vi "rvc Generate Linear Segment with Parabolic Blend.vi"(7 "maximum velocity":dbl=nan, 9 "number of timesteps":dbl, 10 "final position":dbl, 11 "initial position":dbl) -> (0 "error out":errorcluster, 1 "accelaration":cluster{"time":dbl[], "velocity":dbl[]}(graph), 2 "velocity":cluster{"time":dbl[], "velocity":dbl[]}(graph), 3 "position":cluster{"time":dbl[], "position":dbl[]}(graph))   [LabVIEW 2019]
uses:
  <vilib>/Analysis/1siggen.llb/Ramp Pattern by Samples.vi
  <vilib>/Utility/error.llb/Error Cluster From Error Code.vi
  <vilib>/ErrorRing/Error Ring.xnode
  <vilib>/Analysis/NI_AALBase.lvlib
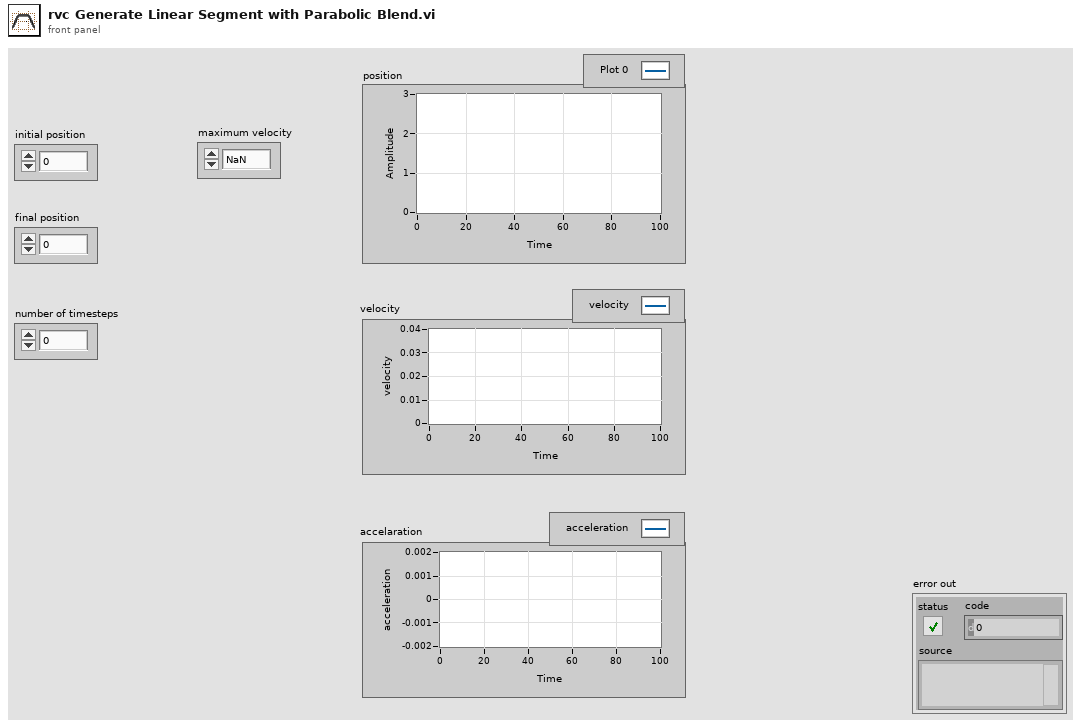
[diagram p1: front panel]
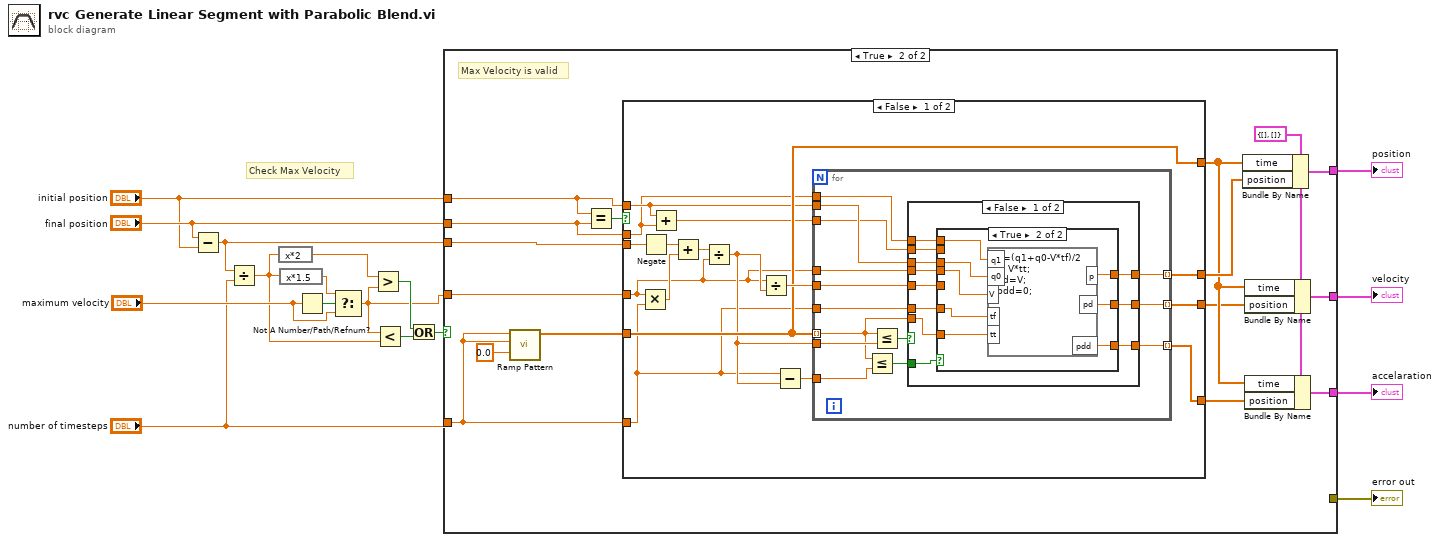
[diagram p0: block diagram]
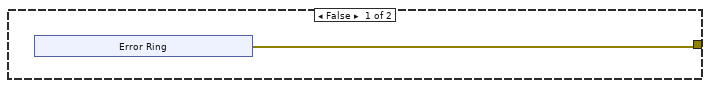
[diagram p2: hidden frame]
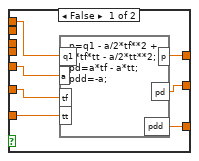
[diagram p3: hidden frame]
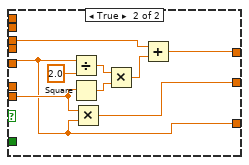
[diagram p4: hidden frame]
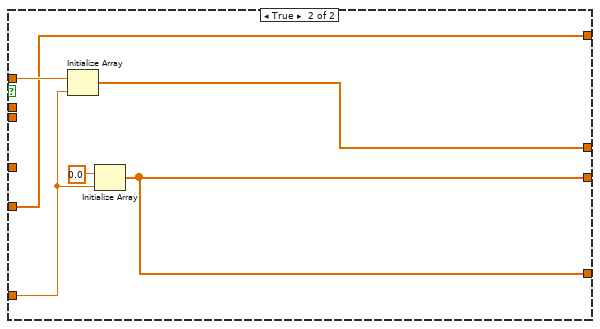
[diagram p5: hidden frame]
diagram:
  # "Check Max Velocity"
  n1 = Subtract(x="final position", y="initial position") -> (x-y=w8:dbl)
  n2 = Divide(x=w8, y="number of timesteps") -> (x/y=w2:dbl)
  n3 = expression code="x*2"(w2) -> (w3:dbl)
  n4 = expression code="x*1.5"(w2) -> (w1:dbl)
  n5 = Not A Number/Path/Refnum?(number/path/refnum="maximum velocity") -> (NaN/Path/Refnum?=w14:bool)
  n6 = Select(t=w1, s=w14, f="maximum velocity") -> (s? t:f=w4:dbl)
  n7 = Greater?(x=w3, y=w4) -> (0:w6:bool)
  n8 = Less?(x=w4, y=w2) -> (x < y?=w5:bool)
  n9 = Or(x=w6, y=w5) -> (x .or. y?=w7:bool)
  n10 = case shown="True" w7 {
    tunnel: [_ w39] -> w17
    tunnel: [_ w38] -> w16
    tunnel: [_ w37] -> w15
    tunnel: "final position" -> [_ w33]
    tunnel: "initial position" -> [_ w36]
    tunnel: "number of timesteps" -> [_ w29]
    tunnel: [w18 _] -> w9
    tunnel: w8 -> [_ w32]
    tunnel: w4 -> [_ w31]
    frame False {
      n11 = xnode "Error Ring"() -> ("error out"=w18:errorcluster)
    }
    frame True {
      w24 = cluster{"time":dbl[], "position":dbl[]} {"time"=[], "position"=[]} ("input cluster")
      # "Max Velocity is valid"
      n12 = call-poly <vilib>:"Ramp Pattern.vi"("start"=0.0, "end"=w29, "samples"=w29) -> ("Ramp Pattern"=w28:dbl[])  [unwired: 7 in, 1 out]
      n13 = Equal?(x=w36, y=w33) -> (x = y?=w34:bool)
      n14 = case shown="False" w34 {
        tunnel: w29 -> [w41 w110]
        tunnel: w36 -> [w43 w109]
        tunnel: [w49 w108] -> w35
        tunnel: [w47 w105] -> w26
        tunnel: w33 -> [w40 _]
        tunnel: w32 -> [w55 _]
        tunnel: w31 -> [w44 _]
        tunnel: w28 -> [w50 w106]
        tunnel: [w50 w106] -> w27
        tunnel: [w48 w105] -> w25
        frame False {
          n15 = Multiply(x=w44, y=w41) -> (x*y=w53:dbl)
          n16 = Negate(x=w55) -> (-x=w54:dbl)
          n17 = Add(x=w43, y=w40) -> (x+y=w42:dbl)
          n18 = Add(x=w54, y=w53) -> (x+y=w52:dbl)
          n19 = Divide(x=w52, y=w44) -> (x/y=w46:dbl)
          n20 = Divide(x=w44, y=w46) -> (x/y=w51:dbl)
          n21 = Subtract(x=w41, y=w46) -> (x-y=w45:dbl)
          n22 = for {
            tunnel: w50 -> [w63] mode=indexing
            tunnel: w51 -> [w66]
            tunnel: w46 -> [w69]
            tunnel: w43 -> [w68]
            tunnel: [w67] -> w49 mode=indexing
            tunnel: [w59] -> w48 mode=indexing
            tunnel: [w65] -> w47 mode=indexing
            tunnel: w45 -> [w62]
            tunnel: w44 -> [w60]
            tunnel: w42 -> [w58]
            tunnel: w41 -> [w57]
            tunnel: w40 -> [w56]
            n23 = Less Or Equal?(x=w63, y=w62) -> (x <= y?=w61:bool)
            n24 = Less Or Equal?(x=w63, y=w69) -> (x <= y?=w64:bool)
            n25 = case shown="False" w64 {
              tunnel: w66 -> [w77 w96]
              tunnel: w68 -> [w70 w104]
              tunnel: w63 -> [w71 w98]
              tunnel: [w73 w99] -> w67
              tunnel: [w78 w97] -> w65
              tunnel: w61 -> [w80 _]
              tunnel: w60 -> [w79 _]
              tunnel: [w76 w96] -> w59
              tunnel: w58 -> [w75 _]
              tunnel: w57 -> [w74 _]
              tunnel: w56 -> [w72 _]
              frame False {
                n26 = case shown="True" w80 {
                  tunnel: w79 -> [_ w89]
                  tunnel: [w83 w92] -> w78
                  tunnel: w77 -> [w86 _]
                  tunnel: [w87 w95] -> w76
                  tunnel: w75 -> [_ _]
                  tunnel: w74 -> [w84 w93]
                  tunnel: [w82 w91] -> w73
                  tunnel: w72 -> [w81 w90]
                  tunnel: w71 -> [w85 w94]
                  tunnel: w70 -> [_ w88]
                  frame False {
                    n27 = formula code="p=q1 - a/2*tf**2 + a*tf*tt - a/2*tt**2;\npd=a*tf - a*tt;\npdd=-a;"("q1"=w81, "a"=w86, "tf"=w84, "tt"=w85) -> ("pdd"=w87:dbl, "p"=w82:dbl, "pd"=w83:dbl)
                  }
                  frame True {
                    n28 = formula code="p=(q1+q0-V*tf)/2 + V*tt;\npd=V;\npdd=0;"("q1"=w90, "V"=w89, "tf"=w93, "tt"=w94, "q0"=w88) -> ("pdd"=w95:dbl, "p"=w91:dbl, "pd"=w92:dbl)
                  }
                }
              }
              frame True {
                n29 = Divide(x=w96, y=2.0) -> (x/y=w102:dbl)
                n30 = Square(x=w98) -> (x^2=w101:dbl)
                n31 = Multiply(x=w98, y=w96) -> (x*y=w97:dbl)
                n32 = Multiply(x=w102, y=w101) -> (x*y=w100:dbl)
                n33 = Add(x=w104, y=w100) -> (x+y=w99:dbl)
              }
            }
          }
        }
        frame True {
          n34 = Initialize Array(w109, w110) -> (w108:dbl[])
          n35 = Initialize Array(0.0 ("element"), w110) -> (w105:dbl[])
        }
      }
      n36 = Bundle By Name(cluster=w24, "time"=w27, "position"=w35) -> (w37:cluster{"time":dbl[], "position":dbl[]})
      n37 = Bundle By Name(cluster=w24, "time"=w27, "position"=w26) -> (w38:cluster{"time":dbl[], "position":dbl[]})
      n38 = Bundle By Name(cluster=w24, "time"=w27, "position"=w25) -> (w39:cluster{"time":dbl[], "position":dbl[]})
    }
  }
  "position" <- w15
  "accelaration" <- w17
  "velocity" <- w16
  "error out" <- w9
